vi "set font.vi"(8 "error in (no error)":errorcluster, 10 "Ring Text.Font":T1, 11 "Ring Control in":refnum<class "Ring Control.lvclass">) -> (0 "error out":errorcluster, 3 "Ring Control out":refnum<class "Ring Control.lvclass">)   [LabVIEW 2010, in "Ring Control.lvclass"]
uses:
  Ring Control.lvclass
  <vilib>/Utility/miscctls.llb/LVFontTypeDef.ctl
  Ring Control.lvclass/Ring Control.ctl
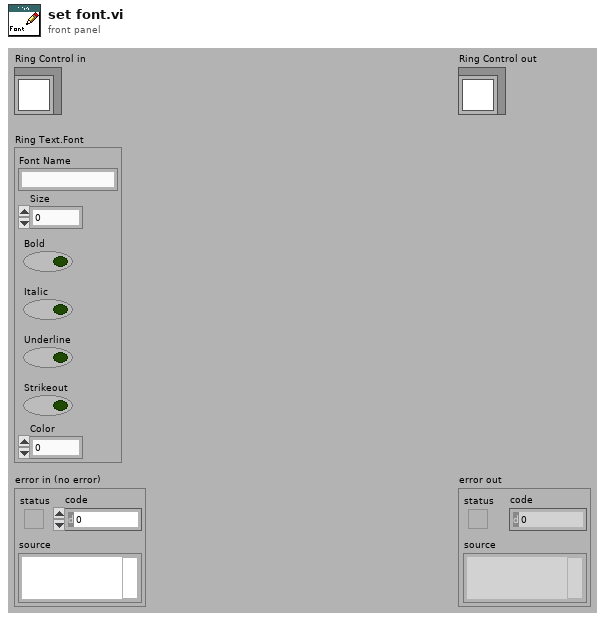
[diagram p1: front panel]
types:
  T1 = typedef "LVFontTypeDef.ctl" = cluster{"Font Name":string, "Size":u16, "Bold":bool, "Italic":bool, "Underline":bool, "Strikeout":bool, "Color":u32}
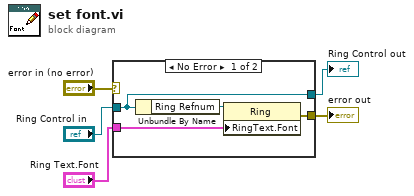
[diagram p0: block diagram]
diagram:
  n1 = case shown="No Error" "error in (no error)" {
    selector: "error in (no error)" -> [_ w11]
    tunnel: [w7 w11] -> w4
    tunnel: [w9 w10] -> w2
    tunnel: "Ring Control in" -> [w9 w10]
    tunnel: "Ring Text.Font" -> [w6 _]
    frame No Error {
      n2 = Unbundle By Name(w9) -> ("Ring Refnum"=w8:refnum<vi>)
      n3 = property class="Ring"(reference=w8, "RingText.Font"=w6) -> (error out=w7:errorcluster)  [unwired: 1 in, 1 out]
    }
    frame Error {
    }
  }
  "error out" <- w4
  "Ring Control out" <- w2
